vi "Read Attributes.vi"(11 "Return IED_Status Msg":refnum<class "Return IED_Status Msg.lvclass">) -> (2 "Payload":cluster{"IED_Status":T1})   [LabVIEW 2018, in "EMS Generic Actor.lvlib" / "Return IED_Status Msg.lvclass"]
uses:
  Return IED_Status Msg.lvclass
  <vilib>/ORNL/CSEISMIC DDS/CSEISMIC DDS Base/Data Types/IED_Status.ctl
  <vilib>/ORNL/CSEISMIC DDS/CSEISMIC DDS Base/Data Types/Controls/DeviceID.ctl
  <vilib>/ORNL/CSEISMIC DDS/CSEISMIC DDS Base/Data Types/Controls/Timestamp.ctl
  Return IED_Status Msg.lvclass/Return IED_Status Msg.ctl
  <vilib>/ORNL/CSEISMIC DDS/CSEISMIC DDS Base/CSEISMIC DDS.lvclass
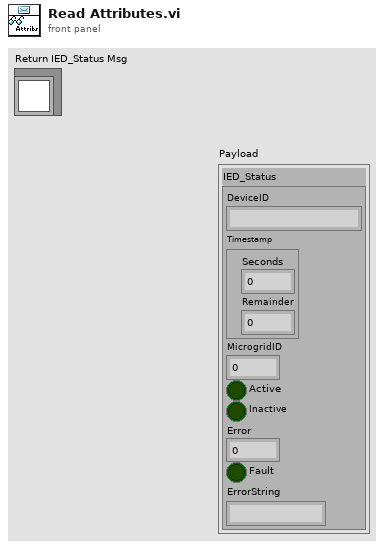
[diagram p1: front panel]
types:
  T1 = typedef "CSEISMIC DDS.lvlib/CSEISMIC DDS.lvclass/IED_Status.ctl" = cluster{"DeviceID":T2, "Timestamp":T3, "MicrogridID":u8, "Active":bool, "Inactive":bool, "Error":i32, "Fault":bool, "ErrorString":string}
  T2 = typedef "CSEISMIC DDS.lvlib/CSEISMIC DDS.lvclass/DeviceID.ctl" = string
  T3 = typedef "CSEISMIC DDS.lvlib/CSEISMIC DDS.lvclass/Timestamp.ctl" = cluster{"Seconds":u64, "Remainder":u64}
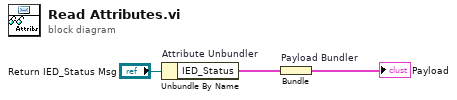
[diagram p0: block diagram]
diagram:
  n1 = Unbundle By Name "Attribute Unbundler"("Return IED_Status Msg") -> ("IED_Status"=w1:T1)
  n2 = Bundle "Payload Bundler"("IED_Status"=w1) -> (→"Payload":cluster{"IED_Status":T1})  [unwired: 1 in]
